vi "TreeNode Get Data.vi"(8 "error in (no error)":errorcluster, 11 "TreeNode DVR in":refnum<data-value>) -> (0 "error out":errorcluster, 2 "Data out":refnum<data-value>, 3 "TreeNode DVR out":refnum<data-value>)   [LabVIEW 2013, in "MDSplus.lvlib"]
doc: "Get Data for this node."
uses:
  <vilib>/MDSplus/Library/MDSplus.lvlib
  <vilib>/MDSplus/Classes/Data_Class/TreeNode_Class/TreeNode.lvclass
  <vilib>/MDSplus/Classes/Data_Class/Data.lvclass
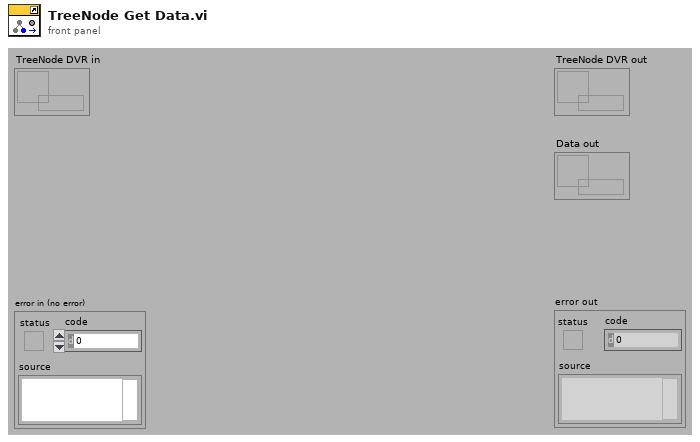
[diagram p1: front panel]
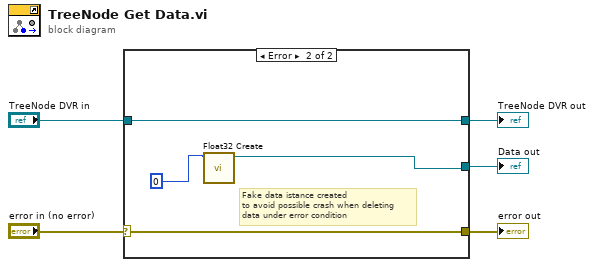
[diagram p0: block diagram]
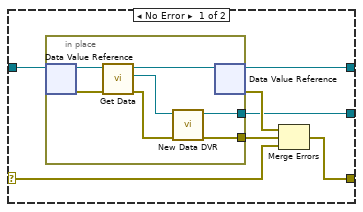
[diagram p2: hidden frame]
diagram:
  n1 = case shown="Error" "error in (no error)" {
    selector: "error in (no error)" -> [w11 w23]
    tunnel: "TreeNode DVR in" -> [w12 w22]
    tunnel: [w8 w23] -> w5
    tunnel: [w9 w22] -> w2
    tunnel: [w6 w20] -> w1
    frame No Error {
      n2 = in-place {
        in-place-border: [w15] -> w6
        in-place-border: [w14] -> w7
        n3 = in-place-dvr #1(w12) -> (w19:refnum<class "TreeNode.lvclass">, w18:errorcluster)
        n4 = call-dynamic "Get Data.vi"("error in (no error)"=w18, "TreeNode in"=w19) -> ("error out"=w13:errorcluster, "Data out"=w16:refnum<class "Data.lvclass">, "TreeNode out"=w17:refnum<class "TreeNode.lvclass">)  [unwired: 7 in]
        n5 = call <vilib>:"New Data DVR.vi"("error in (no error)"=w13, "Data in"=w16) -> ("error out"=w14:errorcluster, "Data DVR out"=w15:refnum<data-value>)  [unwired: 8 in]
        n6 = in-place-dvr #1(w17) -> (w9:refnum<data-value>, w10:errorcluster)
      }
      n7 = Merge Errors(w10, w7, w11) -> (w8:errorcluster)
    }
    frame Error {
      # "Fake data istance created \nto avoid possible crash when deleting\ndata under error condition"
      n8 = call <vilib>:"Float32 Create.vi"("SGL in"=0) -> ("Float32 DVR out"=w20:refnum<data-value>)  [unwired: 9 in, 1 out]
    }
  }
  "error out" <- w5
  "TreeNode DVR out" <- w2
  "Data out" <- w1
